vi "keyboard_control__nxt.vi"() -> ()   [LabVIEW 2012]
uses:
  <vilib>/NXT/Block Support/NXT_MessageMailbox.ctl
  <vilib>/NXT/Block Support/NXT_OutputPort.ctl
  <vilib>/NXT/Subs/MotorOutput.ctl
  <vilib>/NXT/Dual Mode Library/Waits/Wait_BT.vi
  <vilib>/NXT/Dual Mode Library/Display/drawText.vi
  <vilib>/NXT/Dual Mode Library/Display/drawNumber.vi
  <vilib>/NXT/Dual Mode Library/Waits/Wait_Num.vi
  <vilib>/NXT/NXTIO Xnodes/NXTIONodeSubVIs/NXTStopMotors.vi
  <vilib>/NXT/Dual Mode Library/Motors/MotorOn.vi
  <vilib>/NXT/Dual Mode Library/Motors/MotorBrake.vi
  <vilib>/NXT/Dual Mode Library/Motors/MotorReverse.vi
  <vilib>/NXT/NXTIO Xnodes/AddressXNode/NXTIOAddress.xnode
  <vilib>/NXT/NXTIO Xnodes/NXTIOXNode/NXTIO.xnode
  <vilib>/NXT/Subs/LVHSConnector.ctl
  <vilib>/NXT/LegoClasses/BrickReference/BrickReference.lvclass
panel:
  out "status":string
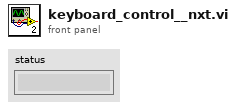
[diagram p1: front panel]
types:
  T1 = typedef "NXT_OutputPort.ctl" = u8
  T2 = typedef "NXT_MessageMailbox.ctl" = u8
  T3 = typedef "LVHSConnector.ctl" = refnum<class "BrickReference.lvclass">
  T4 = typedef "MotorOutput.ctl" = u8
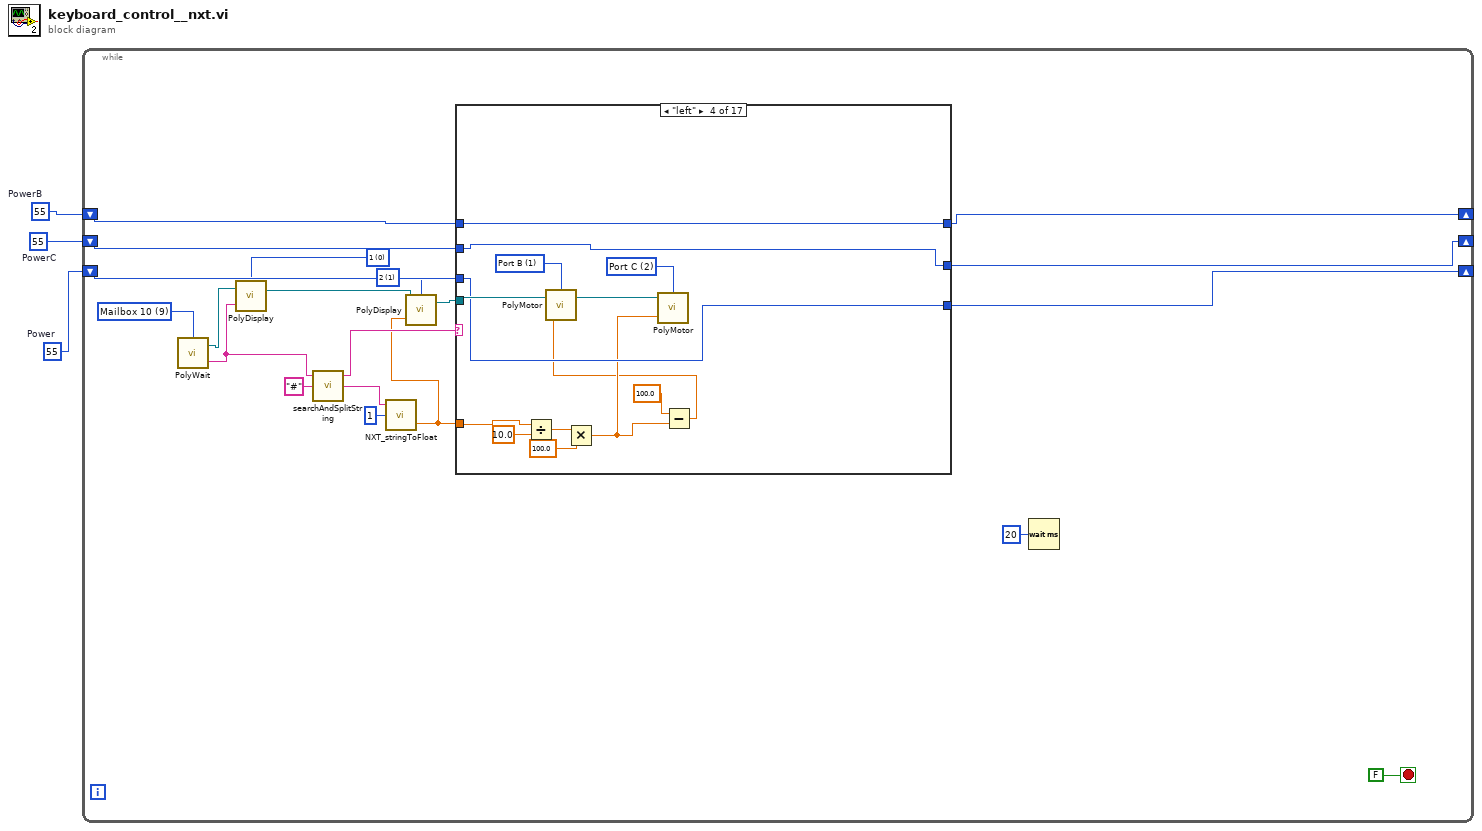
[diagram p0: block diagram]
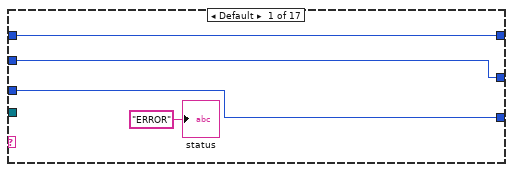
[diagram p2: hidden frame]
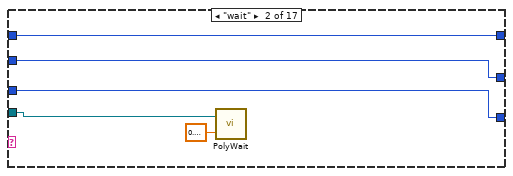
[diagram p3: hidden frame]
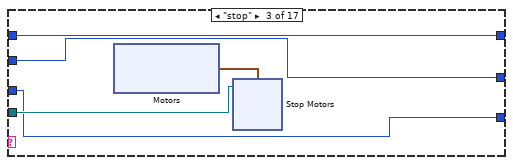
[diagram p4: hidden frame]
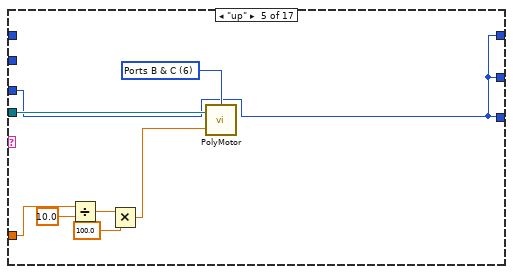
[diagram p5: hidden frame]
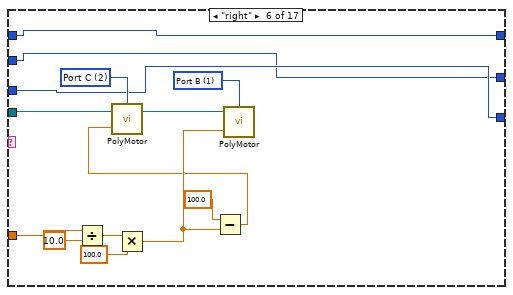
[diagram p6: hidden frame]
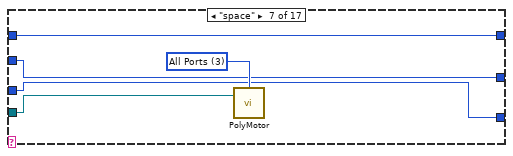
[diagram p7: hidden frame]
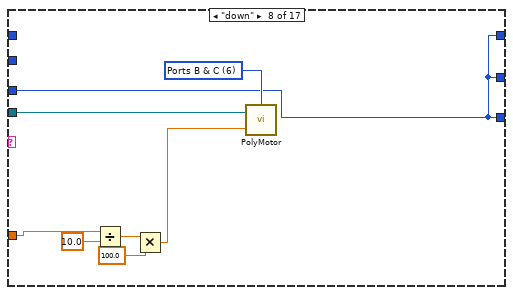
[diagram p8: hidden frame]
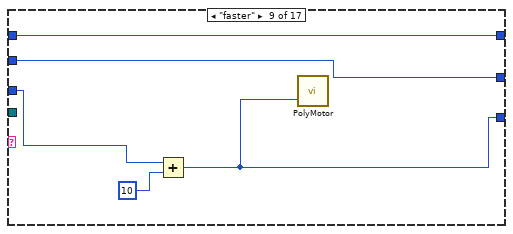
[diagram p9: hidden frame]
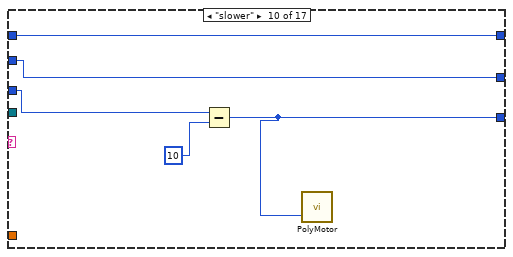
[diagram p10: hidden frame]
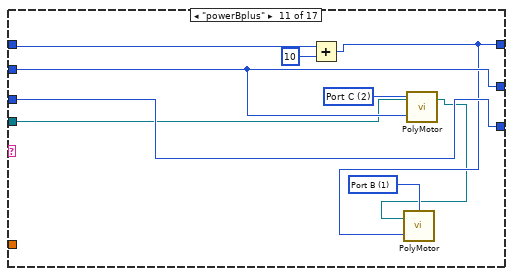
[diagram p11: hidden frame]
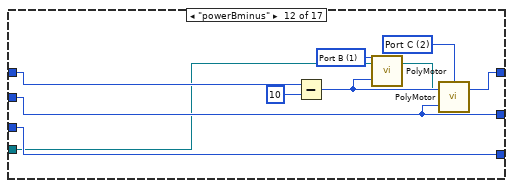
[diagram p12: hidden frame]
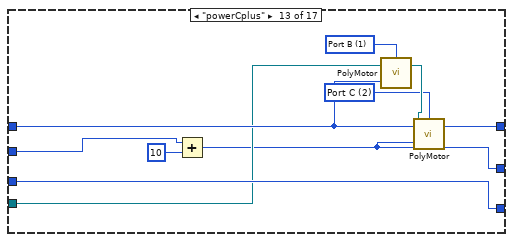
[diagram p13: hidden frame]
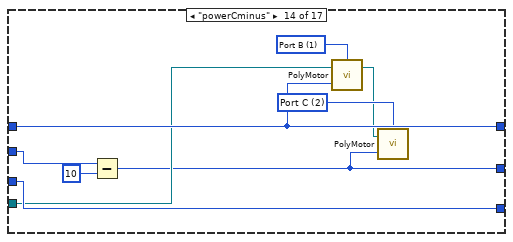
[diagram p14: hidden frame]
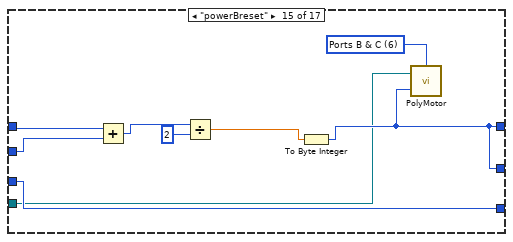
[diagram p15: hidden frame]
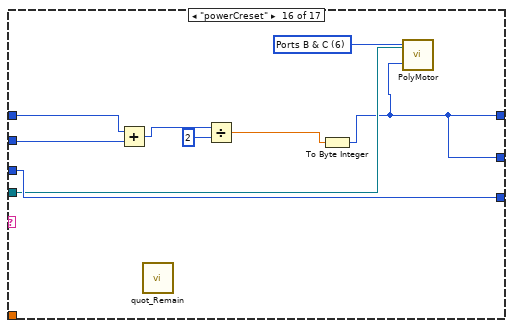
[diagram p16: hidden frame]
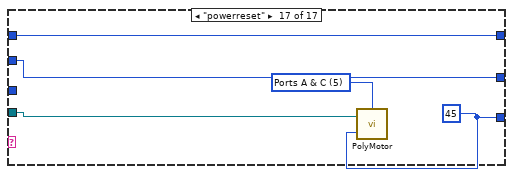
[diagram p17: hidden frame]
diagram:
  w2 = 55  # PowerC
  w1 = 55  # PowerB
  w3 = 55  # Power
  n1 = while {
    shift-right: [w15] -> _
    shift-left: w3 -> [w23]
    shift-right: [w17] -> _
    shift-left: w1 -> [w21]
    shift-right: [w16] -> _
    shift-left: w2 -> [w22]
    stop <- FALSE stop-if-true
    w4 = i16 1 items=["1", "2", "3", "4", "5", "6", "7", "8", "9", "10", "11", "12"] ("Line")
    w18 = i16 0 items=["1", "2", "3", "4", "5", "6", "7", "8", "9", "10", "11", "12"] ("Line")
    w20 = T2 9 items=["Mailbox 1", "Mailbox 2", "Mailbox 3", "Mailbox 4", "Mailbox 5", "Mailbox 6", "Mailbox 7", "Mailbox 8", "Mailbox 9", "Mailbox 10"] ("Mailbox")
    n2 = call-poly <vilib>:"PolyWait.vi"("Mailbox"=w20) -> ("Message"=w9:string, "NXT/EV3"=w19:T3)  [unwired: 2 in]
    n3 = call-poly <vilib>:"PolyDisplay.vi"("Text"=w9, "NXT/EV3"=w19, "Line"=w18) -> ("NXT/EV3"=w11:T3)  [unwired: 1 in]
    n4 = call <vilib>:"searchAndSplitString.vi"("search string/char (-)"="#", "string"=w9) -> ("match + rest of string"=w6:string, "substring before match"=w8:string)  [unwired: 1 in, 1 out]
    n5 = call <vilib>:"NXT_stringToFloat.vi"("offset"=1, "string"=w6) -> ("number"=w5:sgl)  [unwired: 1 in, 1 out]
    n6 = call-poly <vilib>:"PolyDisplay.vi"("number"=w5, "NXT/EV3"=w11, "Line"=w4) -> ("NXT/EV3"=w12:T3)  [unwired: 1 in]
    n7 = case shown="\"left\"" w8 {
      tunnel: w12 -> [_ w31 w36 w54 w64 w76 w83 w91 _ _ w104 w113 w125 w134 w139 w149 w159]
      tunnel: w23 -> [w26 w30 w33 w53 w63 w75 w82 w90 w96 w101 w107 w120 w129 w138 w142 w151 _]
      tunnel: [w26 w30 w33 w53 w63 w75 w82 w90 w95 w100 w107 w120 w129 w138 w142 w151 w157] -> w15
      tunnel: w22 -> [w25 w29 w34 w51 _ w73 w81 _ w94 w99 w106 w115 w127 w137 w146 w152 w160]
      tunnel: w21 -> [w24 w28 w35 w52 _ w74 w80 _ w93 w98 w110 w118 w126 w135 w147 w153 w161]
      tunnel: [w25 w29 w34 w51 w63 w73 w81 w90 w94 w99 w106 w115 w123 w132 w141 w148 w160] -> w16
      tunnel: [w24 w28 w35 w52 w63 w74 w80 w90 w93 w98 w105 w117 w126 w135 w141 w148 w161] -> w17
      tunnel: w5 -> [_ _ _ w46 w62 w69 _ w86 _ _ _ _ _ _ _ _ _]
      frame Default {
        "status" <- "ERROR" ("status")
      }
      frame "wait" {
        n8 = call-poly <vilib>:"PolyWait.vi"("Time (1 sec)"=sgl 0.1, "NXT/EV3"=w31) -> ()  [unwired: 2 in, 1 out]
      }
      frame "stop" {
        n9 = xnode "Motors"() -> ("Motor"=w37:cluster{"Port":T1, "Port":T1})
        n10 = xnode "Stop Motors"("Motors"=w37, "NXT/EV3"=w36) -> ()  [unwired: 1 out]
      }
      frame "left" {
        w56 = T4 1 items=["Port A"=0, "Port B"=1, "Port C"=2, "Ports A & B"=4, "Ports A & C"=5, "Ports B & C"=6, "All Ports"=3] ("Output Port (All Ports)")
        w57 = T4 2 items=["Port A"=0, "Port B"=1, "Port C"=2, "Ports A & B"=4, "Ports A & C"=5, "Ports B & C"=6, "All Ports"=3] ("Output Port (All Ports)")
        n11 = Divide(x=w46, y=sgl 10.0) -> (x/y=w49:sgl)
        n12 = Multiply(x=w49, y=sgl 100.0) -> (x*y=w45:sgl)
        n13 = Subtract(x=sgl 100.0, y=w45) -> (x-y=w44:sgl)
        n14 = call-poly <vilib>:"PolyMotor.vi"("Power (75)"=w44, "NXT/EV3"=w54, "Output Port (All Ports)"=w56) -> ("NXT/EV3"=w55:T3)  [unwired: 1 in]
        n15 = call-poly <vilib>:"PolyMotor.vi"("Power (75)"=w45, "NXT/EV3"=w55, "Output Port (All Ports)"=w57) -> ()  [unwired: 1 in, 1 out]
      }
      frame "up" {
        w65 = T4 6 items=["Port A"=0, "Port B"=1, "Port C"=2, "Ports A & B"=4, "Ports A & C"=5, "Ports B & C"=6, "All Ports"=3] ("Output Port (All Ports)")
        n16 = Divide(x=w62, y=sgl 10.0) -> (x/y=w60:sgl)
        n17 = Multiply(x=w60, y=sgl 100.0) -> (x*y=w58:sgl)
        n18 = call-poly <vilib>:"PolyMotor.vi"("Power (75)"=w58, "NXT/EV3"=w64, "Output Port (All Ports)"=w65) -> ()  [unwired: 1 in, 1 out]
      }
      frame "right" {
        w78 = T4 2 items=["Port A"=0, "Port B"=1, "Port C"=2, "Ports A & B"=4, "Ports A & C"=5, "Ports B & C"=6, "All Ports"=3] ("Output Port (All Ports)")
        w79 = T4 1 items=["Port A"=0, "Port B"=1, "Port C"=2, "Ports A & B"=4, "Ports A & C"=5, "Ports B & C"=6, "All Ports"=3] ("Output Port (All Ports)")
        n19 = Divide(x=w69, y=sgl 10.0) -> (x/y=w71:sgl)
        n20 = Multiply(x=w71, y=sgl 100.0) -> (x*y=w68:sgl)
        n21 = Subtract(x=sgl 100.0, y=w68) -> (x-y=w66:sgl)
        n22 = call-poly <vilib>:"PolyMotor.vi"("Power (75)"=w66, "NXT/EV3"=w76, "Output Port (All Ports)"=w78) -> ("NXT/EV3"=w77:T3)  [unwired: 1 in]
        n23 = call-poly <vilib>:"PolyMotor.vi"("Power (75)"=w68, "NXT/EV3"=w77, "Output Port (All Ports)"=w79) -> ()  [unwired: 1 in, 1 out]
      }
      frame "space" {
        w84 = T4 3 items=["Port A"=0, "Port B"=1, "Port C"=2, "Ports A & B"=4, "Ports A & C"=5, "Ports B & C"=6, "All Ports"=3] ("Port (All Ports)")
        n24 = call-poly <vilib>:"PolyMotor.vi"("NXT/EV3"=w83, "Port (All Ports)"=w84) -> ()  [unwired: 2 in, 1 out]
      }
      frame "down" {
        w92 = T4 6 items=["Port A"=0, "Port B"=1, "Port C"=2, "Ports A & B"=4, "Ports A & C"=5, "Ports B & C"=6, "All Ports"=3] ("Output Port (All Ports)")
        n25 = Divide(x=w86, y=sgl 10.0) -> (x/y=w88:sgl)
        n26 = Multiply(x=w88, y=sgl 100.0) -> (x*y=w85:sgl)
        n27 = call-poly <vilib>:"PolyMotor.vi"("Power (75)"=w85, "NXT/EV3"=w91, "Output Port (All Ports)"=w92) -> ()  [unwired: 1 in, 1 out]
      }
      frame "faster" {
        n28 = Add(x=w96, y=10) -> (x+y=w95:i32)
        n29 = call-poly <vilib>:"PolyMotor.vi"("Power (75)"=w95) -> ()  [unwired: 3 in, 1 out]
      }
      frame "slower" {
        n30 = Subtract(x=w101, y=10) -> (x-y=w100:i32)
        n31 = call-poly <vilib>:"PolyMotor.vi"("Power (75)"=w100) -> ()  [unwired: 3 in, 1 out]
      }
      frame "powerBplus" {
        w108 = T4 2 items=["Port A"=0, "Port B"=1, "Port C"=2, "Ports A & B"=4, "Ports A & C"=5, "Ports B & C"=6, "All Ports"=3] ("Output Port (All Ports)")
        w109 = T4 1 items=["Port A"=0, "Port B"=1, "Port C"=2, "Ports A & B"=4, "Ports A & C"=5, "Ports B & C"=6, "All Ports"=3] ("Output Port (All Ports)")
        n32 = Add(x=w110, y=10) -> (x+y=w105:i32)
        n33 = call-poly <vilib>:"PolyMotor.vi"("Power (75)"=w106, "NXT/EV3"=w104, "Output Port (All Ports)"=w108) -> ("NXT/EV3"=w103:T3)  [unwired: 1 in]
        n34 = call-poly <vilib>:"PolyMotor.vi"("Power (75)"=w105, "NXT/EV3"=w103, "Output Port (All Ports)"=w109) -> ()  [unwired: 1 in, 1 out]
      }
      frame "powerBminus" {
        w112 = T4 2 items=["Port A"=0, "Port B"=1, "Port C"=2, "Ports A & B"=4, "Ports A & C"=5, "Ports B & C"=6, "All Ports"=3] ("Output Port (All Ports)")
        w116 = T4 1 items=["Port A"=0, "Port B"=1, "Port C"=2, "Ports A & B"=4, "Ports A & C"=5, "Ports B & C"=6, "All Ports"=3] ("Output Port (All Ports)")
        n35 = Subtract(x=w118, y=10) -> (x-y=w117:i32)
        n36 = call-poly <vilib>:"PolyMotor.vi"("Power (75)"=w117, "NXT/EV3"=w113, "Output Port (All Ports)"=w116) -> ("NXT/EV3"=w114:T3)  [unwired: 1 in]
        n37 = call-poly <vilib>:"PolyMotor.vi"("Power (75)"=w115, "NXT/EV3"=w114, "Output Port (All Ports)"=w112) -> ()  [unwired: 1 in, 1 out]
      }
      frame "powerCplus" {
        w121 = T4 2 items=["Port A"=0, "Port B"=1, "Port C"=2, "Ports A & B"=4, "Ports A & C"=5, "Ports B & C"=6, "All Ports"=3] ("Output Port (All Ports)")
        w124 = T4 1 items=["Port A"=0, "Port B"=1, "Port C"=2, "Ports A & B"=4, "Ports A & C"=5, "Ports B & C"=6, "All Ports"=3] ("Output Port (All Ports)")
        n38 = Add(x=w127, y=10) -> (x+y=w123:i32)
        n39 = call-poly <vilib>:"PolyMotor.vi"("Power (75)"=w126, "NXT/EV3"=w125, "Output Port (All Ports)"=w124) -> ("NXT/EV3"=w122:T3)  [unwired: 1 in]
        n40 = call-poly <vilib>:"PolyMotor.vi"("Power (75)"=w123, "NXT/EV3"=w122, "Output Port (All Ports)"=w121) -> ()  [unwired: 1 in, 1 out]
      }
      frame "powerCminus" {
        w131 = T4 2 items=["Port A"=0, "Port B"=1, "Port C"=2, "Ports A & B"=4, "Ports A & C"=5, "Ports B & C"=6, "All Ports"=3] ("Output Port (All Ports)")
        w133 = T4 1 items=["Port A"=0, "Port B"=1, "Port C"=2, "Ports A & B"=4, "Ports A & C"=5, "Ports B & C"=6, "All Ports"=3] ("Output Port (All Ports)")
        n41 = Subtract(x=w137, y=10) -> (x-y=w132:i32)
        n42 = call-poly <vilib>:"PolyMotor.vi"("Power (75)"=w135, "NXT/EV3"=w134, "Output Port (All Ports)"=w133) -> ("NXT/EV3"=w130:T3)  [unwired: 1 in]
        n43 = call-poly <vilib>:"PolyMotor.vi"("Power (75)"=w132, "NXT/EV3"=w130, "Output Port (All Ports)"=w131) -> ()  [unwired: 1 in, 1 out]
      }
      frame "powerBreset" {
        w140 = T4 6 items=["Port A"=0, "Port B"=1, "Port C"=2, "Ports A & B"=4, "Ports A & C"=5, "Ports B & C"=6, "All Ports"=3] ("Output Port (All Ports)")
        n44 = Add(x=w147, y=w146) -> (x+y=w145:i32)
        n45 = Divide(x=w145, y=2) -> (x/y=w143:dbl)
        n46 = To Byte Integer(number=w143) -> (8bit integer=w141:i8)
        n47 = call-poly <vilib>:"PolyMotor.vi"("Power (75)"=w141, "NXT/EV3"=w139, "Output Port (All Ports)"=w140) -> ()  [unwired: 1 in, 1 out]
      }
      frame "powerCreset" {
        w150 = T4 6 items=["Port A"=0, "Port B"=1, "Port C"=2, "Ports A & B"=4, "Ports A & C"=5, "Ports B & C"=6, "All Ports"=3] ("Output Port (All Ports)")
        n48 = Add(x=w153, y=w152) -> (x+y=w156:i32)
        n49 = call <vilib>:"quot_Remain.vi"() -> ()  [unwired: 2 in, 2 out]
        n50 = Divide(x=w156, y=2) -> (x/y=w154:dbl)
        n51 = To Byte Integer(number=w154) -> (8bit integer=w148:i8)
        n52 = call-poly <vilib>:"PolyMotor.vi"("Power (75)"=w148, "NXT/EV3"=w149, "Output Port (All Ports)"=w150) -> ()  [unwired: 1 in, 1 out]
      }
      frame "powerreset" {
        w158 = T4 5 items=["Port A"=0, "Port B"=1, "Port C"=2, "Ports A & B"=4, "Ports A & C"=5, "Ports B & C"=6, "All Ports"=3] ("Output Port (All Ports)")
        w157 = 45 ("Power")
        n53 = call-poly <vilib>:"PolyMotor.vi"("Power (75)"=w157, "NXT/EV3"=w159, "Output Port (All Ports)"=w158) -> ()  [unwired: 1 in, 1 out]
      }
    }
    n54 = Wait (ms)(milliseconds to wait=u32 20) -> ()  [unwired: 1 out]
  }
